vi "ТекстЗапись.vi"() -> ()   [LabVIEW 2017]
panel:
  in  "text":string
  in  "file (use dialog)":path
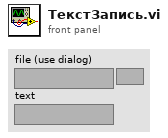
[diagram p1: front panel]
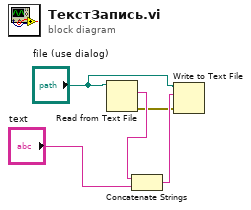
[diagram p0: block diagram]
diagram:
  n1 = Read from Text File(file (use dialog)="file (use dialog)") -> (text=w3:string, error out=w1:errorcluster)  [unwired: 3 in, 2 out]
  n2 = Concatenate Strings(w3, "text") -> (w4:string)
  n3 = Write to Text File(file (use dialog)="file (use dialog)", text=w4, error in=w1) -> ()  [unwired: 1 in, 3 out]
